vi "Auton File Control.vi"(10 "Manip D-Pad":T1, 11 "Manip Button":T2) -> ()   [LabVIEW 2015]
uses:
  Common Code/Gamepads/Button Cluster.ctl
  Common Code/Gamepads/D-Pad.ctl
  Common Code/Change Detect Int.vi
  Common Code/Change Detect Boolean.vi
  Robot Global Data.vi
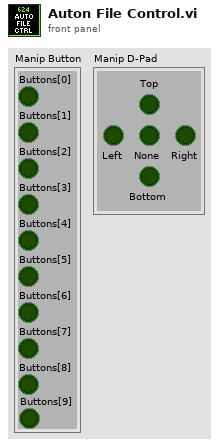
[diagram p1: front panel]
types:
  T1 = typedef "D-Pad.ctl" = cluster{"Top":bool, "Bottom":bool, "None":bool, "Right":bool, "Left":bool}
  T2 = typedef "Button Cluster.ctl" = cluster{"Buttons[0]":bool, "Buttons[1]":bool, "Buttons[2]":bool, "Buttons[3]":bool, "Buttons[4]":bool, "Buttons[5]":bool, "Buttons[6]":bool, "Buttons[7]":bool, "Buttons[8]":bool, "Buttons[9]":bool}
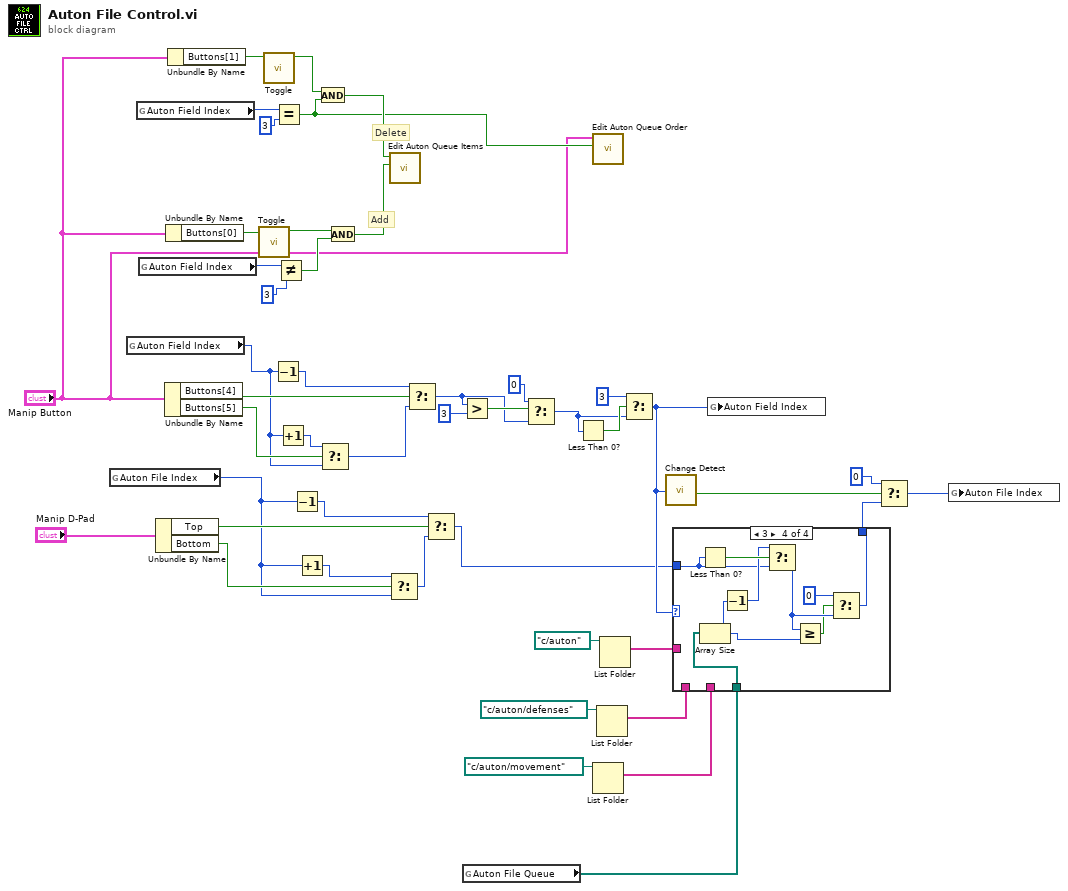
[diagram p0: block diagram]
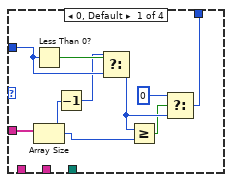
[diagram p2: hidden frame]
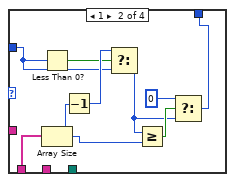
[diagram p3: hidden frame]
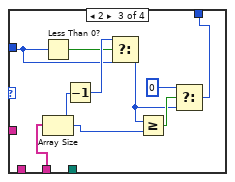
[diagram p4: hidden frame]
diagram:
  # "Delete"
  # "Add"
  n1 = global read "Robot Global Data.vi" "Auton File Index"() -> (w27:i32)
  n2 = global read "Robot Global Data.vi" "Auton Field Index"() -> (w42:i32)
  n3 = global read "Robot Global Data.vi" "Auton Field Index"() -> (w13:i32)
  n4 = global read "Robot Global Data.vi" "Auton Field Index"() -> (w10:i32)
  n5 = Unbundle By Name("Manip D-Pad") -> ("Top"=w29:bool, "Bottom"=w28:bool)
  n6 = Unbundle By Name("Manip Button") -> ("Buttons[4]"=w46:bool, "Buttons[5]"=w44:bool)
  n7 = Unbundle By Name("Manip Button") -> ("Buttons[0]"=w6:bool)
  n8 = Unbundle By Name("Manip Button") -> ("Buttons[1]"=w8:bool)
  n9 = call "Toggle.vi"("In"=w6) -> ("Toggled"=w5:bool)  [unwired: 10 in]
  n10 = call "Toggle.vi"("In"=w8) -> ("Toggled"=w7:bool)  [unwired: 10 in]
  n11 = Decrement(x=w42) -> (x-1=w45:i32)
  n12 = Equal?(x=w13, y=3) -> (x = y?=w2:bool)
  n13 = Not Equal?(x=w10, y=3) -> (x != y?=w9:bool)
  n14 = Increment(x=w42) -> (x+1=w43:i32)
  n15 = Decrement(x=w27) -> (x-1=w30:i32)
  n16 = Increment(x=w27) -> (x+1=w31:i32)
  n17 = And(x=w7, y=w2) -> (x .and. y?=w4:bool)
  n18 = Select(t=w43, s=w44, f=w42) -> (s? t:f=w41:i32)
  n19 = And(x=w5, y=w9) -> (x .and. y?=w3:bool)
  n20 = Select(t=w31, s=w28, f=w27) -> (s? t:f=w32:i32)
  n21 = call "Edit Auton Queue Items.vi"("Add?"=w3, "Delete?"=w4) -> ()  [unwired: 10 in]
  n22 = Select(t=w45, s=w46, f=w41) -> (s? t:f=w38:i32)
  n23 = Select(t=w30, s=w29, f=w32) -> (s? t:f=w22:i32)
  n24 = Greater?(x=w38, y=3) -> (0:w39:bool)
  n25 = global read "Robot Global Data.vi" "Auton File Queue"() -> (w18:path[])
  n26 = Select(t=0, s=w39, f=w38) -> (s? t:f=w35:i32)
  n27 = Less Than 0?(x=w35) -> (x < 0?=w36:bool)
  n28 = call "Edit Auton Queue Order.vi"("Boolean"=w2, "Manip Button"="Manip Button") -> ()  [unwired: 10 in]
  n29 = List Folder(path=path "c/auton/movement") -> (filenames=w19:string[])  [unwired: 3 in, 3 out]
  n30 = List Folder(path=path "c/auton/defenses") -> (filenames=w20:string[])  [unwired: 3 in, 3 out]
  n31 = List Folder(path=path "c/auton") -> (filenames=w21:string[])  [unwired: 3 in, 3 out]
  n32 = Select(t=3, s=w36, f=w35) -> (s? t:f=w23:i32)
  n33 = call-poly "Change Detect.vi"("In"=w23) -> ("Changed?"=w17:bool)
  n34 = case shown="3" w23 {
    tunnel: w22 -> [w53 w57 w66 w75]
    tunnel: w21 -> [w55 _ _ _]
    tunnel: w20 -> [_ w58 _ _]
    tunnel: w19 -> [_ _ w67 _]
    tunnel: w18 -> [_ _ _ w74]
    tunnel: [w47 w56 w65 w76] -> w16
    frame 0, Default {
      n35 = Less Than 0?(x=w53) -> (x < 0?=w54:bool)
      n36 = Array Size(array=w55) -> (size(s)=w50:i32)
      n37 = Decrement(x=w50) -> (x-1=w52:i32)
      n38 = Select(t=w52, s=w54, f=w53) -> (s? t:f=w51:i32)
      n39 = Greater Or Equal?(x=w51, y=w50) -> (x >= y?=w49:bool)
      n40 = Select(t=0, s=w49, f=w51) -> (s? t:f=w47:i32)
    }
    frame 1 {
      n41 = Less Than 0?(x=w57) -> (x < 0?=w59:bool)
      n42 = Array Size(array=w58) -> (size(s)=w62:i32)
      n43 = Decrement(x=w62) -> (x-1=w60:i32)
      n44 = Select(t=w60, s=w59, f=w57) -> (s? t:f=w61:i32)
      n45 = Greater Or Equal?(x=w61, y=w62) -> (x >= y?=w63:bool)
      n46 = Select(t=0, s=w63, f=w61) -> (s? t:f=w56:i32)
    }
    frame 2 {
      n47 = Less Than 0?(x=w66) -> (x < 0?=w68:bool)
      n48 = Array Size(array=w67) -> (size(s)=w71:i32)
      n49 = Decrement(x=w71) -> (x-1=w69:i32)
      n50 = Select(t=w69, s=w68, f=w66) -> (s? t:f=w70:i32)
      n51 = Greater Or Equal?(x=w70, y=w71) -> (x >= y?=w72:bool)
      n52 = Select(t=0, s=w72, f=w70) -> (s? t:f=w65:i32)
    }
    frame 3 {
      n53 = Less Than 0?(x=w75) -> (x < 0?=w82:bool)
      n54 = Array Size(array=w74) -> (size(s)=w79:i32)
      n55 = Decrement(x=w79) -> (x-1=w81:i32)
      n56 = Select(t=w81, s=w82, f=w75) -> (s? t:f=w80:i32)
      n57 = Greater Or Equal?(x=w80, y=w79) -> (x >= y?=w78:bool)
      n58 = Select(t=0, s=w78, f=w80) -> (s? t:f=w76:i32)
    }
  }
  n59 = global write "Robot Global Data.vi" "Auton Field Index"(w23) -> ()
  n60 = Select(t=0, s=w17, f=w16) -> (s? t:f=w14:i32)
  n61 = global write "Robot Global Data.vi" "Auton File Index"(w14) -> ()
